vi "Write.EngineData.vi"(8 "error in":errorcluster, 11 "Write in":refnum<class "Write.lvclass">) -> (0 "error out":errorcluster, 3 "Write out":refnum<class "Write.lvclass">)   [LabVIEW 2015, in "Data Access Engine.lvlib" / "Write.lvclass"]
uses:
  Write.lvclass
  Write.lvclass/Write.ctl
  <vilib>/NI Veristand/Custom Device API/Global Data Refs.vi
  <vilib>/NI Veristand/Custom Device API/Custom Device API.lvlib
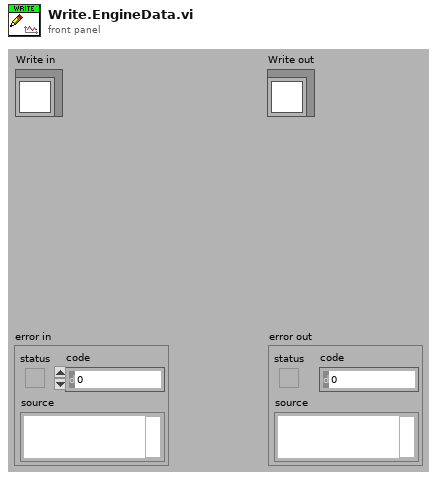
[diagram p1: front panel]
types:
  T1 = typedef "Custom Device API.lvlib/Data Reference.ctl" = i32
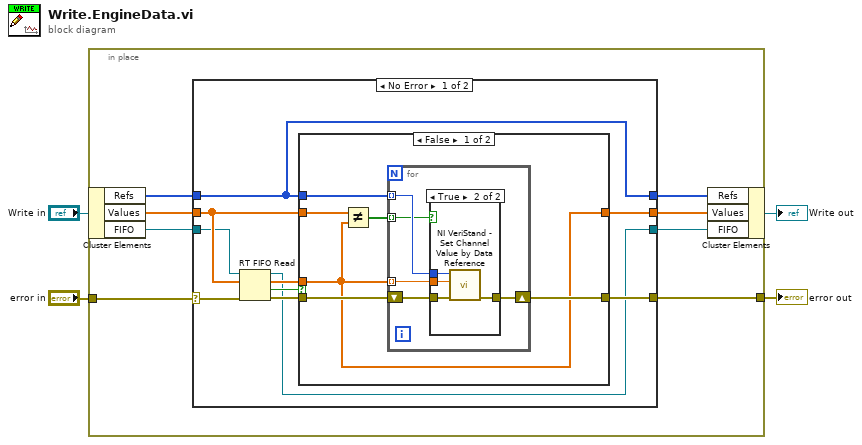
[diagram p0: block diagram]
diagram:
  n1 = in-place {
    in-place-border: [w12] -> w4
    in-place-border: "error in" -> [w7]
    n2 = in-place-cluster #1("Write in") -> ("Refs"=w11:T1[], "Values"=w10:dbl[], "FIFO"=w6:refnum<k33>)
    n3 = case shown="No Error" w7 {
      selector: w7 -> [w19 w44]
      tunnel: [w22 w44] -> w12
      tunnel: [w16 w43] -> w9
      tunnel: w11 -> [w15 w42]
      tunnel: w10 -> [w17 w43]
      tunnel: [w15 w42] -> w8
      tunnel: w6 -> [w14 w41]
      tunnel: [w13 w41] -> w5
      frame No Error {
        n4 = RT FIFO Read(0:w14, 1:w17, 3:w19) -> (8:w13:refnum<k33>, 9:w20:dbl[], 10:w18:bool, 11:w21:errorcluster)  [unwired: 1 in, 1 out]
        n5 = case shown="False" w18 {
          tunnel: w21 -> [w28 w40]
          tunnel: w20 -> [w23 _]
          tunnel: [w27 w40] -> w22
          tunnel: [w23 w39] -> w16
          tunnel: w15 -> [w26 _]
          tunnel: w17 -> [w24 w39]
          frame False {
            n6 = Not Equal?(x=w24, y=w23) -> (x != y?=w25:bool[])
            n7 = for {
              shift-right: [w33] -> w27
              shift-left: w28 -> [w32]
              tunnel: w25 -> [w29] mode=indexing
              tunnel: w23 -> [w31] mode=indexing
              tunnel: w26 -> [w30] mode=indexing
              n8 = case shown="True" w29 {
                tunnel: w31 -> [_ w35]
                tunnel: [w34 w37] -> w33
                tunnel: w32 -> [w34 w38]
                tunnel: w30 -> [_ w36]
                frame False {
                }
                frame True {
                  n9 = call <vilib>:"NI VeriStand - Set Channel Value by Data Reference.vi"("error in (no error)"=w38, "Value"=w35, "Data Reference in"=w36) -> ("error out"=w37:errorcluster)  [unwired: 8 in]
                }
              }
            }
          }
          frame True {
          }
        }
      }
      frame Error {
      }
    }
    n10 = in-place-cluster #1("Refs"=w8, "Values"=w9, "FIFO"=w5) -> (→"Write out":refnum<class "Write.lvclass">)
  }
  "error out" <- w4
